vi "TDTSyn-Init Synapse State.vi"(0 "Settings":T1={"Server IP Address"=4925, "TCP Port"=4925, "Synapse URL"="", "Tank Root"=""}, 11 "error in (no error)":errorcluster) -> (4 "Settings (thru)":T1={"Server IP Address"=4925, "TCP Port"=4925, "Synapse URL"="", "Tank Root"=""}, 8 "State":T2, 15 "error out":errorcluster)   [LabVIEW 2020]
uses:
  TDTSyn-State.ctl
  TDTSyn-Settings.ctl
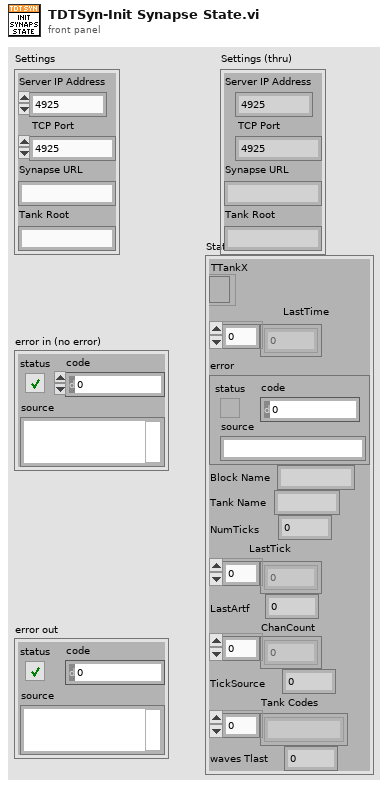
[diagram p1: front panel]
types:
  T1 = typedef "TDTSyn-Settings.ctl" = cluster{"Server IP Address":u32, "TCP Port":u16, "Synapse URL":string, "Tank Root":string}
  T2 = typedef "TDTSyn-State.ctl" = cluster{"TTankX":refnum<k7>, "LastTime":dbl[], "error":errorcluster, "Block Name":string, "Tank Name":string, "NumTicks":i32, "LastTick":dbl[], "LastArtf":dbl, "ChanCount":i32[], "TickSource":i32, "Tank Codes":string[], "waves Tlast":dbl}
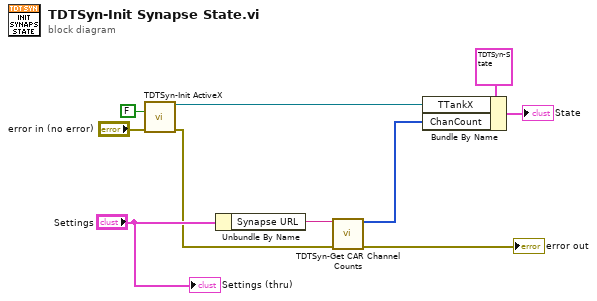
[diagram p0: block diagram]
diagram:
  n1 = call "TDTSyn-Init ActiveX.vi"("Init TDevAccX?"=FALSE, "error in (no error)"="error in (no error)") -> ("TTANKXLib.TTankX"=w9:refnum<k7>, "error out"=w3:errorcluster)  [unwired: 11 in, 1 out]
  n2 = Unbundle By Name("Settings") -> ("Synapse URL"=w4:string)
  n3 = call "TDTSyn-Get CAR Channel Counts.vi"("Synapse URL"=w4, "error in (no error)"=w3) -> ("Channel counts"=w2:i32[], "error out"=→"error out":errorcluster)  [unwired: 12 in]
  n4 = Bundle By Name(cluster=T2 {"TTankX"=refnum, "LastTime"=[], "error"={"status"=FALSE, "code"=0, "source"=""}, "Block Name"="", "Tank Name"="", "NumTicks"=0, "LastTick"=[], "LastArtf"=0.0, "ChanCount"=[], "TickSource"=0, "Tank Codes"=[], "waves Tlast"=0.0} ("State"), "TTankX"=w9, "ChanCount"=w2) -> (→"State":T2)
  "Settings (thru)" <- "Settings"
